vi "Filter Control Key Down.vi"(8 "error in (no error)":errorcluster, 10 "Ctl Refnum":refnum<vi>, 11 "IControlShortcutMenu In":T1) -> (0 "error out":errorcluster, 2 "Discarded?":bool)   [LabVIEW 2015, in "ActorEvents.lvlib" / "IControlKeyDownFilter.lvclass"]
uses:
  IControlKeyDownFilter.lvclass
  ControlKeyDownFilter Reference.ctl
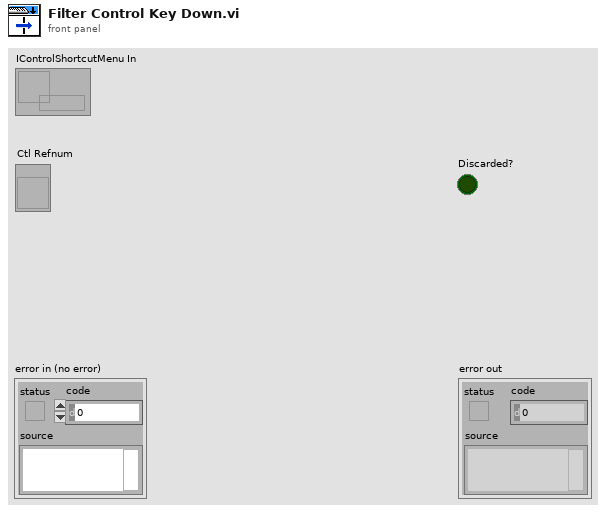
[diagram p1: front panel]
types:
  T1 = typedef "ActorEvents.lvlib/IControlKeyDownFilter.lvclass/ControlKeyDownFilter Reference.ctl" = refnum<data-value>
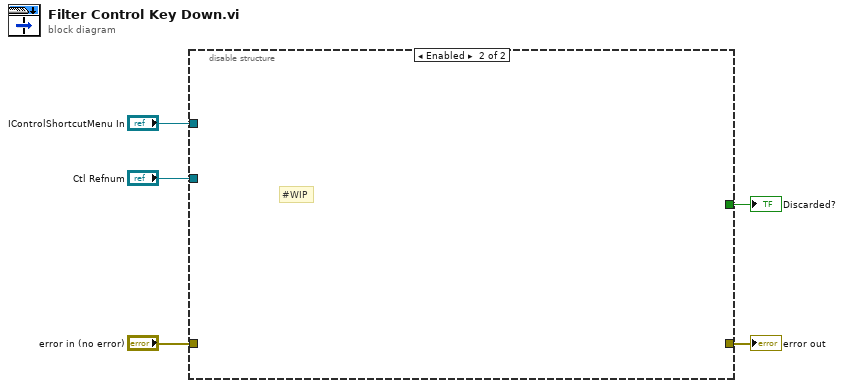
[diagram p0: block diagram]
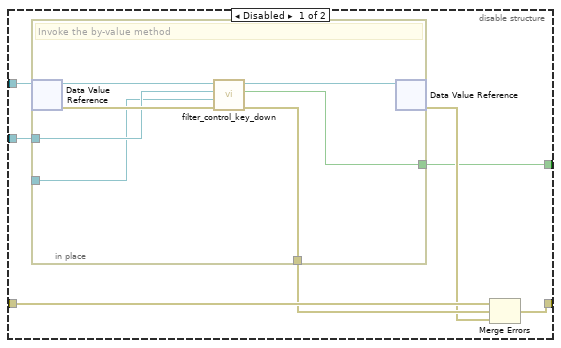
[diagram p2: hidden frame]
diagram:
  n1 = disable-structure shown="Enabled" {
    disable-tunnel: "error in (no error)" -> [w13 _]
    disable-tunnel: "IControlShortcutMenu In" -> [w12 _]
    disable-tunnel: "Ctl Refnum" -> [w11 _]
    disable-tunnel: [w9 _] -> w2
    disable-tunnel: [w6 _] -> w1
    frame Disabled {
      n2 = in-place {
        in-place-border: w11 -> [w15]
        in-place-border: [w14] -> w10
        in-place-border: [w17] -> w8
        in-place-border: [w16] -> w6
        # "Invoke the by-value method"
        n3 = in-place-dvr #1(w12) -> (w20:refnum<class "IControlKeyDownFilter.lvclass">, w18:errorcluster)
        n4 = call-dynamic "filter_control_key_down.vi"("error in (no error)"=w18, 9:w14, "Ctl Refnum"=w15, "IControlShortcutMenu In"=w20) -> ("error out"=w17:errorcluster, "Discarded?"=w16:bool, "IControlShortcutMenu Out"=w19:refnum<class "IControlKeyDownFilter.lvclass">)  [unwired: 5 in]
        n5 = in-place-dvr #1(w19) -> (w7:errorcluster)  [unwired: 1 out]
      }
      n6 = Merge Errors(w13, w8, w7) -> (w9:errorcluster)
    }
    frame Enabled {
      # "#WIP"
    }
  }
  "error out" <- w2
  "Discarded?" <- w1
